vi "Close Audio.vi"(8 "error in":errorcluster) -> (0 "error out":errorcluster)   [LabVIEW 2015, in "LibSDL2_Mixer.lvlib"]
uses:
  LibSDL2_Mixer.lvlib
  LibSDL2 Wrapper/DLL/SDL2_mixer.dll
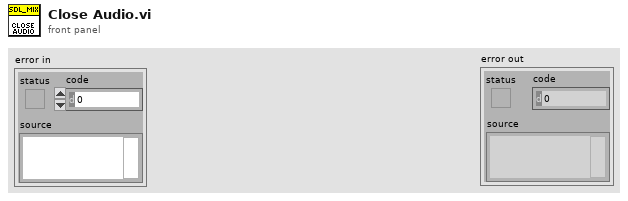
[diagram p1: front panel]
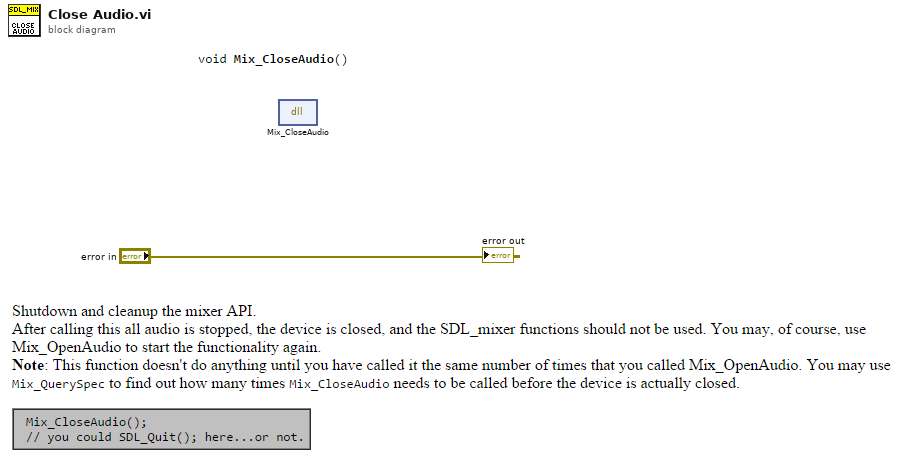
[diagram p0: block diagram]
diagram:
  n1 = dll-call lib="C:/dev/PGS/LabSDL2/Source/Libraries/LibSDL2 Wrapper/DLL/SDL2_mixer.dll" fn="Mix_CloseAudio"() -> ()  [unwired: 4 in, 2 out]
  "error out" <- "error in"
